vi "Teleop.vi"() -> ()   [LabVIEW 2016]
doc: "This VI is called for each TeleOp packet received from the DS where the robot is not disabled. It is often used to read from the joysticks and update I/O or to update setpoints for timed control loops. It should complete and return within 20 milliseconds or it may miss DS packets."
uses:
  <vilib>/Rock Robotics/WPI/ThirdParty/CanMotor/TalonSRX/WPI_CANTalonSRX_APIControlMode.ctl
  <vilib>/Rock Robotics/WPI/Joystick/WPI_JoystickDeviceEnum.ctl
panel:
  in  "stop":bool
  out "X-Value":dbl
  out "Y-Value":dbl
  out "X-Value 2":dbl
  out "Y-Value 2":dbl
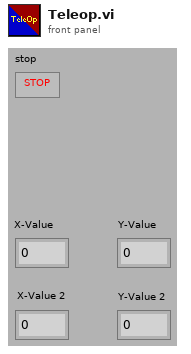
[diagram p1: front panel]
types:
  T1 = typedef "WPI_JoystickDeviceEnum.ctl" = enum16{"USB 0", "USB 1", "USB 2", "USB 3", "USB 4", "USB 5"}
  T2 = typedef "WPI_CANTalonSRX_APIControlMode.ctl" = enum8{"Percent VBus", "Speed", "Position", "Slave", "Unchanged / Invalid", "Voltage Compensation", "Current", "Motion Profile", "Motion Magic"}
  T3 = typedef "WPI_MotorControlDeviceRef.ctl" = cluster{"DeviceStatus":errorcluster, "Type":T4, "PWM":cluster{"PWM Channel":T5, "DeadBand":T6}, "CAN":cluster{"Device Number":u8, "SetOutput VI Ref":variant, "GetOutput VI Ref":variant, "Enable VI Ref":variant, "Disable VI Ref":variant, "Data":variant}, "Invert":bool}
  T4 = typedef "WPI_MotorControlType.ctl" = enum16{"PWM", "CAN"}
  T5 = typedef "FPGA_DIOPWMChannel.ctl" = enum8{"PWM 0", "PWM 1", "PWM 2", "PWM 3", "PWM 4", "PWM 5", "PWM 6", "PWM 7", "PWM 8", "PWM 9", "PWM MXP 0", "PWM MXP 1", "PWM MXP 2", "PWM MXP 3", "PWM MXP 4", "PWM MXP 5", "PWM MXP 6", "PWM MXP 7", "PWM MXP 8", "PWM MXP 9", "Invalid"}
  T6 = typedef "WPI_PWMDeadband.ctl" = cluster{"Name":string, "maxPositivePwm":i32, "minPositivePwm":i32, "centerPwm":i32, "maxNegativePwm":i32, "minNegativePwm":i32, "angularRange":u16}
  T7 = typedef "WPI_JoystickDevRef.ctl" = cluster{"Device":T1}
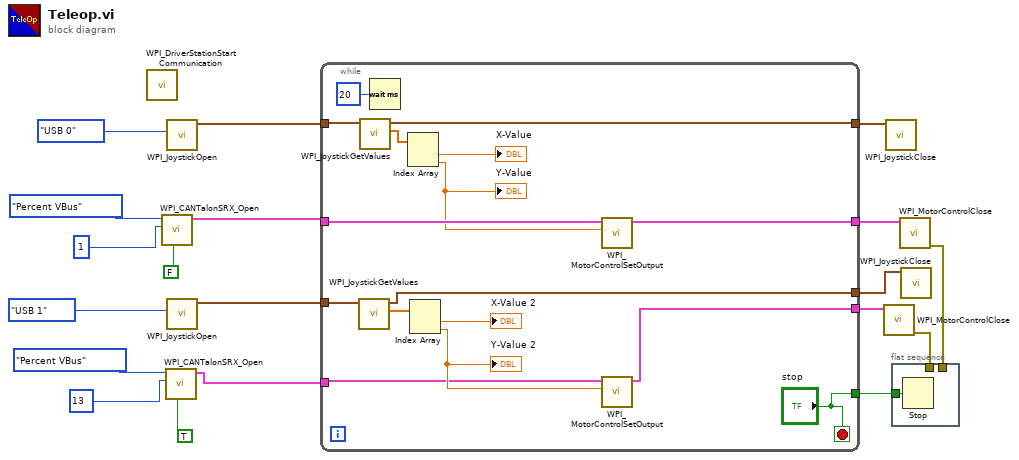
[diagram p0: block diagram]
diagram:
  n1 = call <vilib>:"WPI_DriverStationStart Communication.vi"() -> ()  [unwired: 12 in]
  n2 = call <vilib>:"WPI_CANTalonSRX_Open.vi"("Invert"=FALSE, "Device Number"=u8 1, "Control Mode"=WPI_CANTalonSRX_APIControlMode."Percent VBus") -> ("CAN Talon SRX Ref"=w11:T3)  [unwired: 7 in, 1 out]
  n3 = call <vilib>:"WPI_CANTalonSRX_Open.vi"("Invert"=TRUE, "Device Number"=u8 13, "Control Mode"=WPI_CANTalonSRX_APIControlMode."Percent VBus") -> ("CAN Talon SRX Ref"=w6:T3)  [unwired: 7 in, 1 out]
  n4 = call <vilib>:"WPI_JoystickOpen.vi"("JoystickDevice"=WPI_JoystickDeviceEnum."USB 0") -> ("JoystickDevRef"=w19:T7)  [unwired: 10 in]
  n5 = call <vilib>:"WPI_JoystickOpen.vi"("JoystickDevice"=WPI_JoystickDeviceEnum."USB 1") -> ("JoystickDevRef"=w15:T7)  [unwired: 10 in]
  n6 = while {
    tunnel: w19 -> [w22]
    tunnel: [w21] -> w18
    tunnel: ["stop"] -> w17
    tunnel: w11 -> [w33]
    tunnel: [w32] -> w16
    tunnel: w15 -> [w30]
    tunnel: w6 -> [w23]
    tunnel: [w26] -> w14
    tunnel: [w25] -> w3
    stop <- "stop" stop-if-true
    n7 = call <vilib>:"WPI_JoystickGetValues.vi"("JoystickDevRef"=w30) -> ("Axes"=w29:dbl[], "JoystickDevRef"=w25:T7)  [unwired: 6 in, 3 out]
    n8 = call <vilib>:"WPI_JoystickGetValues.vi"("JoystickDevRef"=w22) -> ("Axes"=w20:dbl[], "JoystickDevRef"=w21:T7)  [unwired: 6 in, 3 out]
    n9 = Wait (ms)(milliseconds to wait=u32 20) -> ()  [unwired: 1 out]
    n10 = Index Array(array=w20) -> (element #1=→"X-Value":dbl, element #2=w27:dbl)  [unwired: 2 in]
    "Y-Value" <- w27
    n11 = Index Array(array=w29) -> (element #1=→"X-Value 2":dbl, element #2=w24:dbl)  [unwired: 2 in]
    "Y-Value 2" <- w24
    n12 = call <vilib>:"WPI_MotorControlSetOutput.vi"("Output"=w27, "MotorControlDevRef"=w33) -> ("MotorControlDevRef"=w32:T3)  [unwired: 7 in, 2 out]
    n13 = call <vilib>:"WPI_MotorControlSetOutput.vi"("Output"=w24, "MotorControlDevRef"=w23) -> ("MotorControlDevRef"=w26:T3)  [unwired: 7 in, 2 out]
  }
  n14 = call <vilib>:"WPI_MotorControlClose.vi"("MotorControlDevRef"=w14) -> ("error out"=w12:errorcluster)  [unwired: 10 in]
  n15 = call <vilib>:"WPI_JoystickClose.vi"("JoystickDevRef"=w18) -> ()  [unwired: 11 in]
  n16 = flat-sequence {
    tunnel: w17 -> [w36]
    tunnel: w13 -> [_]
    tunnel: w12 -> [_]
    frame #0 {
      n17 = Stop(stop? (T)=w36) -> ()
    }
  }
  n18 = call <vilib>:"WPI_MotorControlClose.vi"("MotorControlDevRef"=w16) -> ("error out"=w13:errorcluster)  [unwired: 10 in]
  n19 = call <vilib>:"WPI_JoystickClose.vi"("JoystickDevRef"=w3) -> ()  [unwired: 11 in]
